vi "sub_TabloBoya.vi"(2 "Table in":refnum<vi>, 3 "Tablo Degerleri":dbl[][](array[numeric])) -> (0 "Test Result":bool, 1 "RESULTS":string[](array[string]))   [LabVIEW 2014]
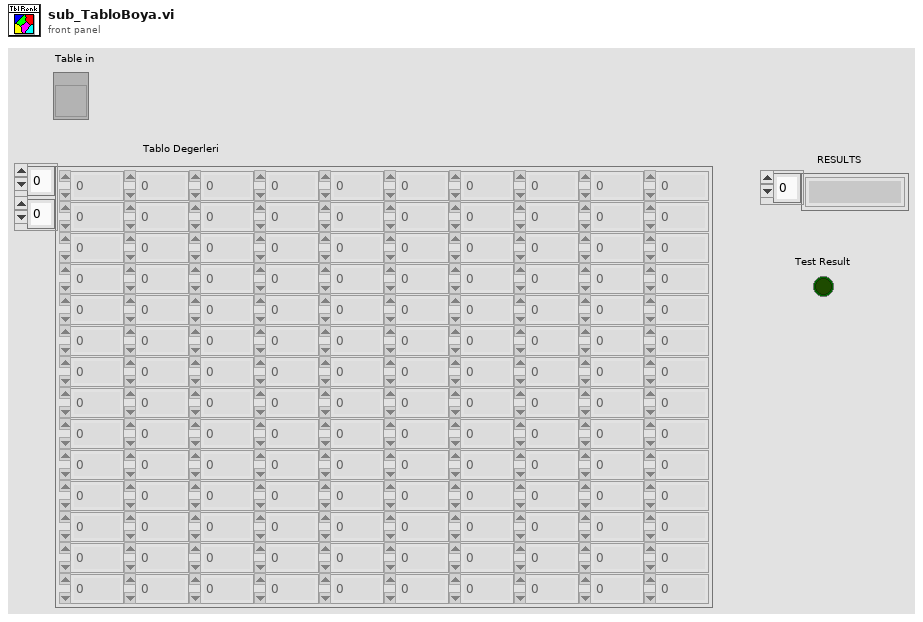
[diagram p1: front panel]
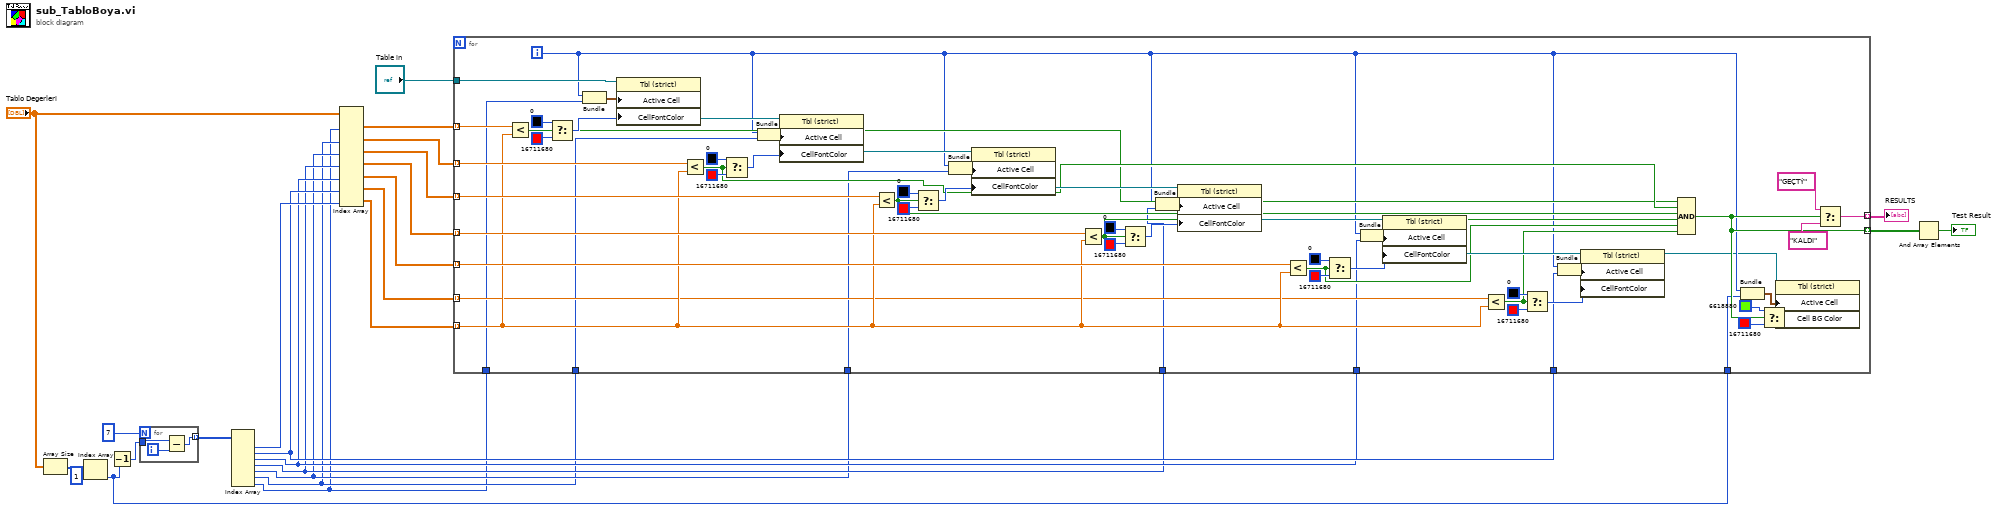
[diagram p0: block diagram]
diagram:
  n1 = Array Size(array="Tablo Degerleri") -> (size(s)=w13:i32[])
  n2 = Index Array(array=w13, index=1) -> (element=w7:i32)
  n3 = Decrement(x=w7) -> (x-1=w8:i32)
  n4 = for {
    N: 7 -> [_]
    tunnel: [w26] -> w11 mode=indexing
    tunnel: w8 -> [w27]
    i -> [w28]
    n5 = Subtract(x=w27, y=w28) -> (x-y=w26:i32)
  }
  n6 = Index Array(array=w11) -> (element #1=w9:i32, element #2=w6:i32, element #3=w5:i32, element #4=w4:i32, element #5=w3:i32, element #6=w2:i32, element #7=w1:i32)  [unwired: 7 in]
  n7 = Index Array(array="Tablo Degerleri", index (col) #1=w1, index (col) #2=w2, index (col) #3=w3, index (col) #4=w4, index (col) #5=w5, index (col) #6=w6, index (col) #7=w9) -> (element #1=w23:dbl[], element #2=w22:dbl[], element #3=w24:dbl[], element #4=w21:dbl[], element #5=w20:dbl[], element #6=w19:dbl[], element #7=w18:dbl[])  [unwired: 7 in]
  n8 = for {
    tunnel: "Table in" -> [w85]
    tunnel: w24 -> [w71] mode=indexing
    tunnel: w23 -> [w83] mode=indexing
    tunnel: w22 -> [w77] mode=indexing
    tunnel: w21 -> [w65] mode=indexing
    tunnel: w20 -> [w59] mode=indexing
    tunnel: w19 -> [w52] mode=indexing
    tunnel: w18 -> [w53] mode=indexing
    tunnel: [w43] -> w17 mode=indexing
    tunnel: [w42] -> w16 mode=indexing
    tunnel: w7 -> [w35]
    tunnel: w6 -> [w34]
    tunnel: w5 -> [w33]
    tunnel: w4 -> [w32]
    tunnel: w3 -> [w31]
    tunnel: w2 -> [w29]
    tunnel: w1 -> [w30]
    i -> [w38]
    n9 = Less?(x=w83, y=w53) -> (x < y?=w46:bool)
    n10 = Select(t=u32 0, s=w46, f=u32 16711680) -> (s? t:f=w86:u32)
    n11 = Bundle(w38, w30) -> (w84:cluster{i32, i32})  [unwired: 1 in]
    n12 = property on="Property Node" class="Tbl (strict)"(reference=w85, "Active Cell"=w84, "CellFontColor"=w86) -> (reference out=w78:refnum<vi>)  [unwired: 1 in, 1 out]
    n13 = Less?(x=w77, y=w53) -> (x < y?=w47:bool)
    n14 = Select(t=u32 0, s=w47, f=u32 16711680) -> (s? t:f=w81:u32)
    n15 = Bundle(w38, w29) -> (w82:cluster{i32, i32})  [unwired: 1 in]
    n16 = property on="Property Node" class="Tbl (strict)"(reference=w78, "Active Cell"=w82, "CellFontColor"=w81) -> (reference out=w72:refnum<vi>)  [unwired: 1 in, 1 out]
    n17 = Less?(x=w71, y=w53) -> (x < y?=w48:bool)
    n18 = Select(t=u32 0, s=w48, f=u32 16711680) -> (s? t:f=w74:u32)
    n19 = Bundle(w38, w31) -> (w73:cluster{i32, i32})  [unwired: 1 in]
    n20 = property on="Property Node" class="Tbl (strict)"(reference=w72, "Active Cell"=w73, "CellFontColor"=w74) -> (reference out=w66:refnum<vi>)  [unwired: 1 in, 1 out]
    n21 = Less?(x=w65, y=w53) -> (x < y?=w49:bool)
    n22 = Select(t=u32 0, s=w49, f=u32 16711680) -> (s? t:f=w68:u32)
    n23 = Bundle(w38, w32) -> (w67:cluster{i32, i32})  [unwired: 1 in]
    n24 = property on="Property Node" class="Tbl (strict)"(reference=w66, "Active Cell"=w67, "CellFontColor"=w68) -> (reference out=w60:refnum<vi>)  [unwired: 1 in, 1 out]
    n25 = Less?(x=w59, y=w53) -> (x < y?=w50:bool)
    n26 = Select(t=u32 0, s=w50, f=u32 16711680) -> (s? t:f=w62:u32)
    n27 = Bundle(w38, w33) -> (w61:cluster{i32, i32})  [unwired: 1 in]
    n28 = property on="Property Node" class="Tbl (strict)"(reference=w60, "Active Cell"=w61, "CellFontColor"=w62) -> (reference out=w54:refnum<vi>)  [unwired: 1 in, 1 out]
    n29 = Less?(x=w52, y=w53) -> (x < y?=w51:bool)
    n30 = Select(t=u32 0, s=w51, f=u32 16711680) -> (s? t:f=w56:u32)
    n31 = Bundle(w38, w34) -> (w55:cluster{i32, i32})  [unwired: 1 in]
    n32 = property on="Property Node" class="Tbl (strict)"(reference=w54, "Active Cell"=w55, "CellFontColor"=w56) -> (reference out=w36:refnum<vi>)  [unwired: 1 in, 1 out]
    n33 = Compound Arithmetic op=AND(w46, w47, w48, w49, w50, w51) -> (w42:bool)
    n34 = Bundle(w38, w35) -> (w37:cluster{i32, i32})  [unwired: 1 in]
    n35 = Select(t=u32 6618880, s=w42, f=u32 16711680) -> (s? t:f=w39:u32)
    n36 = property on="Property Node" class="Tbl (strict)"(reference=w36, "Active Cell"=w37, "Cell BG Color"=w39) -> ()  [unwired: 1 in, 2 out]
    n37 = Select(t="GEÇTÝ", s=w42, f="KALDI") -> (s? t:f=w43:string)
  }
  "RESULTS" <- w17
  n38 = And Array Elements(Boolean array=w16) -> (logical AND=→"Test Result":bool)
